vi "Send Message and Wait for Response.vi"(7 "Message Priority (Normal)":T1=enum."Normal", 8 "error in":errorcluster, 9 "Reply Protocol DataSocket in":refnum<class "Reply Protocol DataSocket.lvclass">, 10 "Original Message":refnum<class "Reply Msg DataSocket.lvclass">, 11 "Message Enqueuer in":refnum<class "Message Enqueuer.lvclass">) -> (0 "error out":errorcluster, 1 "Timeout?":bool, 2 "Reply":variant, 3 "Message Enqueuer out":refnum<class "Message Enqueuer.lvclass">)   [LabVIEW 2023, in "Reply Msg DataSocket.lvclass"]
uses:
  Reply Msg DataSocket.lvclass
  HAL/HAL GOOP4/Reply Protocol/Reply Protocol DataSocket/Reply Protocol DataSocket.lvclass
  <vilib>/ActorFramework/Message Enqueuer/Message Enqueuer.lvclass
  <vilib>/ActorFramework/Message Enqueuer/Message Priority.ctl
  HAL/HAL GOOP4/Reply Protocol/Reply Protocol Base/Reply Protocol Base.lvclass/Reply Protocol Base.ctl
  Reply Msg DataSocket.lvclass/Reply Msg DataSocket.ctl
  <vilib>/ActorFramework/Message Enqueuer/Message Enqueuer.lvclass/Message Enqueuer.ctl
  <vilib>/ActorFramework/Message Priority Queue/Priority Enqueue.vi
  HAL/HAL GOOP4/Reply Protocol/Reply Protocol Base/Reply Protocol Base.lvclass
  D:/git/HAL/HAL GOOP4/Reply Protocol/Reply Protocol Base/Reply Protocol Base.lvclass
  D:/git/HAL/HAL GOOP4/Reply Protocol/Reply Protocol DataSocket/Reply Protocol DataSocket.lvclass
  C:/Program Files/National Instruments/LabVIEW 2023/vi.lib/ActorFramework/Message/Message.lvclass
  D:/git/Reply-Msg-DataSocket/Reply Msg DS/Reply Msg DataSocket.lvclass
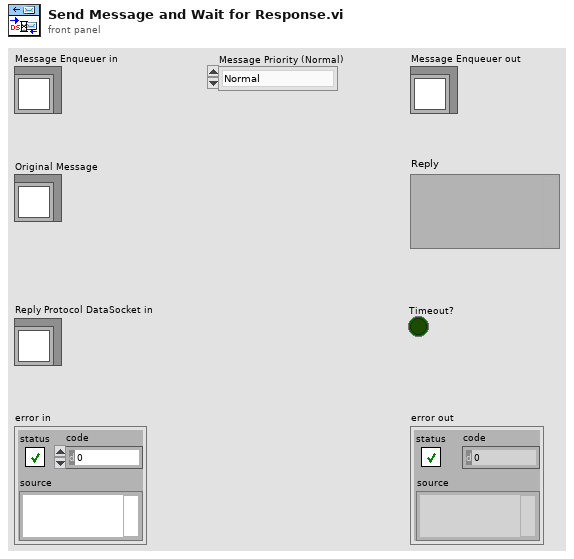
[diagram p1: front panel]
types:
  T1 = typedef "Actor Framework.lvlib/Message Enqueuer.lvclass/Message Priority.ctl" = enum16{"Low", "Normal", "High"}
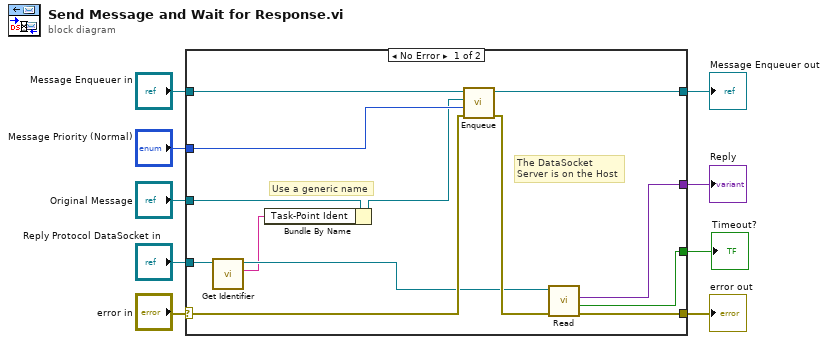
[diagram p0: block diagram]
diagram:
  n1 = case shown="No Error" "error in" {
    selector: "error in" -> [w13 w24]
    tunnel: [w17 w24] -> w4
    tunnel: "Original Message" -> [w19 _]
    tunnel: "Message Enqueuer in" -> [w22 w23]
    tunnel: [w16 _] -> w7
    tunnel: "Message Priority (Normal)" -> [w21 _]
    tunnel: [w20 w23] -> w6
    tunnel: "Reply Protocol DataSocket in" -> [w15 _]
    tunnel: [w14 _] -> w1
    frame No Error {
      # "Use a generic name"
      # "The DataSocket\nServer is on the Host"
      n2 = call "Get Identifier.vi"("Reply Protocol Base in"=w15) -> ("Identifier"=w10:string, "Reply Protocol Base out"=w12:refnum<class "Reply Protocol DataSocket.lvclass">)  [unwired: 9 in]
      n3 = Bundle By Name(cluster=w19, "Task-Point Ident"=w10) -> (w11:refnum<class "Reply Msg DataSocket.lvclass">)
      n4 = call <vilib>:"Enqueue.vi"("error in (no error)"=w13, "Message Priority (Normal)"=w21, "Message"=w11, "Message Enqueuer in"=w22) -> ("error out"=w18:errorcluster, "Message Enqueuer in"=w20:refnum<class "Message Enqueuer.lvclass">)  [unwired: 6 in]
      n5 = call-dynamic "Read.vi"("error in"=w18, "Reply Protocol DataSocket in"=w12) -> ("error out"=w17:errorcluster, "Timeout?"=w14:bool, "Reply"=w16:variant)  [unwired: 6 in, 1 out]
    }
    frame Error {
    }
  }
  "error out" <- w4
  "Reply" <- w7
  "Message Enqueuer out" <- w6
  "Timeout?" <- w1
